vi "选择条件，选择函数的 练习.vi"() -> ()   [LabVIEW 2023]
panel:
  out "选择条件运行时间":dbl
  out "选择函数运行时间":dbl
  out "s? t:f":dbl
  in  "String 3":string
  out "Numeric 2":dbl
  in  "String 2":string
  out "x*y":dbl
  in  "stop":bool
  out "时间长度":dbl
  out "迭代次数":i32
  in  "Numeric":i32
  # "选择条件，选择函数的 练习"
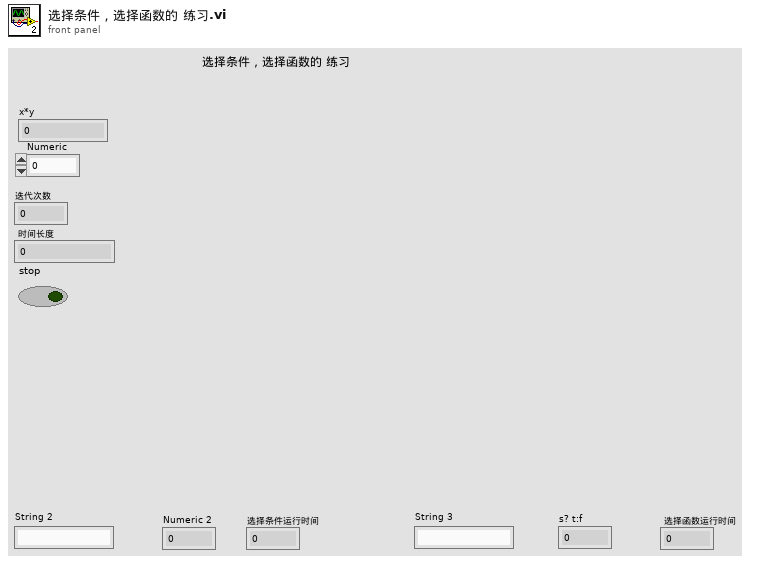
[diagram p1: front panel]
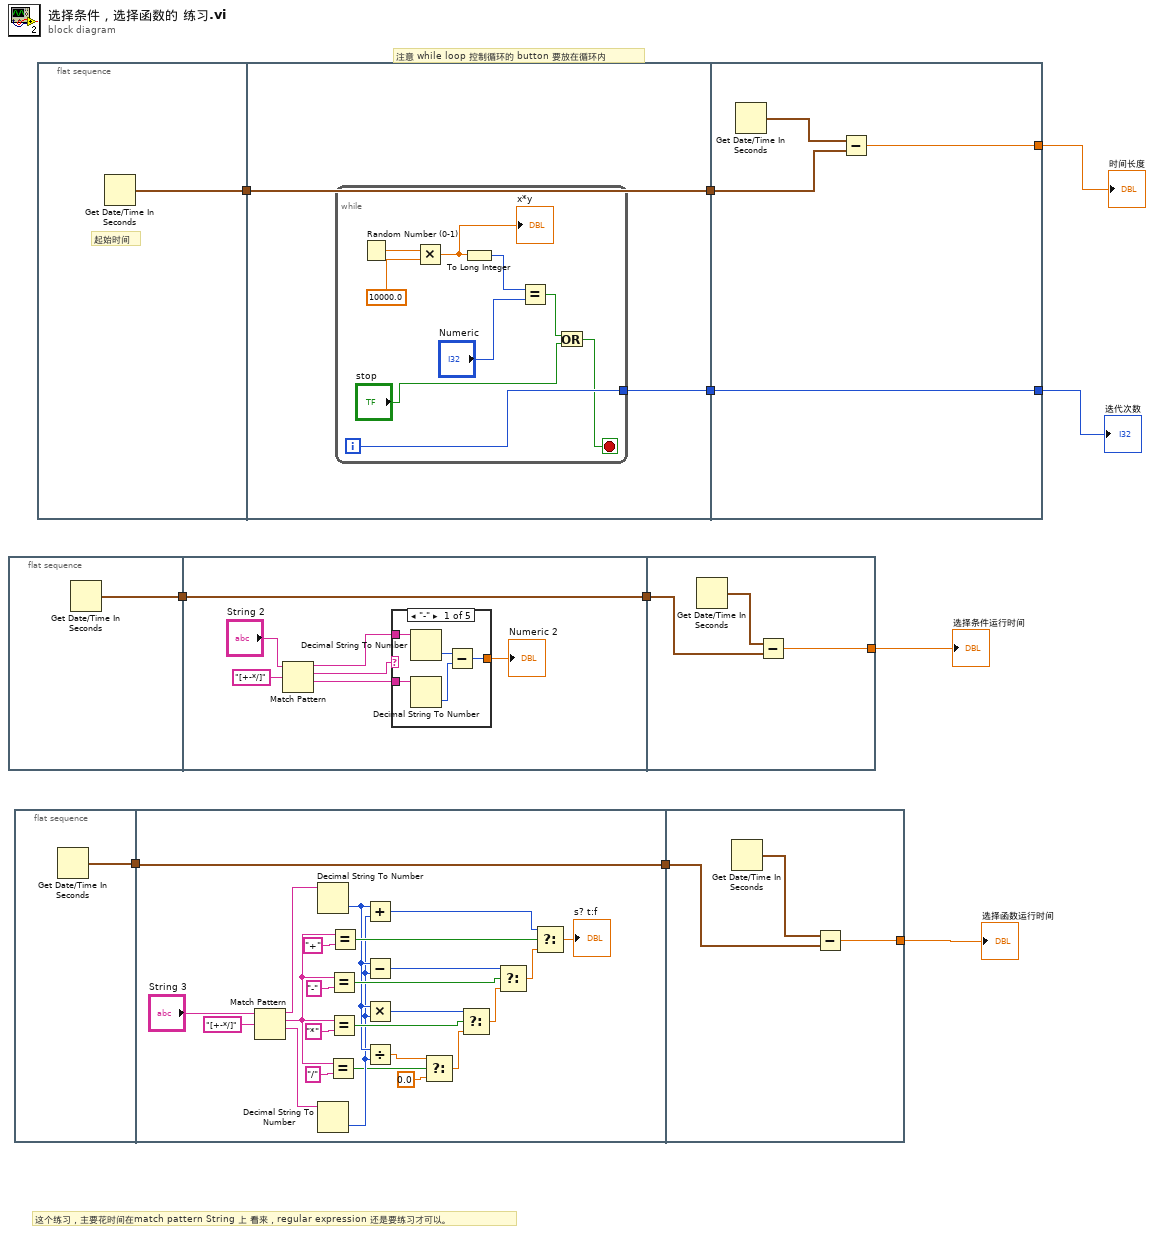
[diagram p0: block diagram]
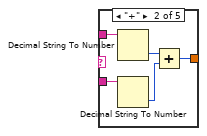
[diagram p2: hidden frame]
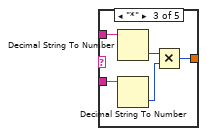
[diagram p3: hidden frame]
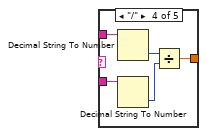
[diagram p4: hidden frame]
diagram:
  # "这个练习，主要花时间在match pattern String 上 看来，regular expression 还是要练习才可以。"
  # "注意 while loop 控制循环的 button 要放在循环内"
  n1 = flat-sequence {
    tunnel: [w12] -> w6
    tunnel: w6 -> [w13]
    tunnel: [w13] -> w2
    tunnel: w2 -> [w41]
    tunnel: [w40] -> w1
    frame #0 {
      n2 = Get Date/Time In Seconds() -> (seconds since 1Jan1904=w12:timestamp)
    }
    frame #1 {
      n3 = Match Pattern(string="String 2", regular expression="[+-*/]") -> (before substring=w16:string, match substring=w17:string, after substring=w15:string)  [unwired: 1 in, 1 out]
      n4 = case shown="\"-\"" w17 {
        tunnel: w16 -> [w24 w29 w34 w39 _]
        tunnel: w15 -> [w23 w28 w33 w38 _]
        tunnel: [w20 w25 w30 w35 _] -> w14
        frame "-" {
          n5 = Decimal String To Number(string=w24) -> (number=w22:i32)  [unwired: 2 in, 1 out]
          n6 = Decimal String To Number(string=w23) -> (number=w21:i32)  [unwired: 2 in, 1 out]
          n7 = Subtract(x=w22, y=w21) -> (x-y=w20:i32)
        }
        frame "+" {
          n8 = Decimal String To Number(string=w29) -> (number=w27:i32)  [unwired: 2 in, 1 out]
          n9 = Decimal String To Number(string=w28) -> (number=w26:i32)  [unwired: 2 in, 1 out]
          n10 = Add(x=w27, y=w26) -> (x+y=w25:i32)
        }
        frame "*" {
          n11 = Decimal String To Number(string=w34) -> (number=w32:i32)  [unwired: 2 in, 1 out]
          n12 = Decimal String To Number(string=w33) -> (number=w31:i32)  [unwired: 2 in, 1 out]
          n13 = Multiply(x=w32, y=w31) -> (x*y=w30:i32)
        }
        frame "/" {
          n14 = Decimal String To Number(string=w39) -> (number=w37:i32)  [unwired: 2 in, 1 out]
          n15 = Decimal String To Number(string=w38) -> (number=w36:i32)  [unwired: 2 in, 1 out]
          n16 = Divide(x=w37, y=w36) -> (x/y=w35:dbl)
        }
        frame Default {
        }
      }
      "Numeric 2" <- w14
    }
    frame #2 {
      n17 = Get Date/Time In Seconds() -> (seconds since 1Jan1904=w42:timestamp)
      n18 = Subtract(x=w42, y=w41) -> (x-y=w40:dbl)
    }
  }
  n19 = flat-sequence {
    tunnel: [w43] -> w5
    tunnel: w5 -> [w44]
    tunnel: [w44] -> w4
    tunnel: w4 -> [w70]
    tunnel: [w69] -> w3
    frame #0 {
      n20 = Get Date/Time In Seconds() -> (seconds since 1Jan1904=w43:timestamp)
    }
    frame #1 {
      n21 = Match Pattern(string="String 3", regular expression="[+-*/]") -> (before substring=w65:string, match substring=w52:string, after substring=w64:string)  [unwired: 1 in, 1 out]
      n22 = Decimal String To Number(string=w65) -> (number=w50:i32)  [unwired: 2 in, 1 out]
      n23 = Decimal String To Number(string=w64) -> (number=w49:i32)  [unwired: 2 in, 1 out]
      n24 = Equal?(x=w52, y="/") -> (x = y?=w47:bool)
      n25 = Equal?(x=w52, y="-") -> (x = y?=w59:bool)
      n26 = Equal?(x=w52, y="*") -> (x = y?=w54:bool)
      n27 = Equal?(x=w52, y="+") -> (x = y?=w63:bool)
      n28 = Add(x=w50, y=w49) -> (x+y=w62:i32)
      n29 = Subtract(x=w50, y=w49) -> (x-y=w58:i32)
      n30 = Multiply(x=w50, y=w49) -> (x*y=w55:i32)
      n31 = Divide(x=w50, y=w49) -> (x/y=w48:dbl)
      n32 = Select(t=w48, s=w47, f=0.0) -> (s? t:f=w53:dbl)
      n33 = Select(t=w55, s=w54, f=w53) -> (s? t:f=w57:dbl)
      n34 = Select(t=w58, s=w59, f=w57) -> (s? t:f=w60:dbl)
      n35 = Select(t=w62, s=w63, f=w60) -> (s? t:f=→"s? t:f":dbl)
    }
    frame #2 {
      n36 = Get Date/Time In Seconds() -> (seconds since 1Jan1904=w71:timestamp)
      n37 = Subtract(x=w71, y=w70) -> (x-y=w69:dbl)
    }
  }
  n38 = flat-sequence {
    tunnel: [w72] -> w11
    tunnel: w11 -> [w73]
    tunnel: [w74] -> w10
    tunnel: [w73] -> w8
    tunnel: [w87] -> w9
    tunnel: w10 -> [w87]
    tunnel: w8 -> [w85]
    tunnel: [w84] -> w7
    frame #0 {
      # "起始时间"
      n39 = Get Date/Time In Seconds() -> (seconds since 1Jan1904=w72:timestamp)
    }
    frame #1 {
      n40 = while {
        tunnel: [w80] -> w74
        i -> [w80]
        stop <- w78 stop-if-true
        n41 = Random Number (0-1)() -> (number: 0 to 1=w83:dbl)
        n42 = Multiply(x=w83, y=10000.0) -> (x*y=w76:dbl)
        "x*y" <- w76
        n43 = To Long Integer(number=w76) -> (32bit integer=w77:i32)
        n44 = Equal?(x=w77, y="Numeric") -> (x = y?=w79:bool)
        n45 = Or(x=w79, y="stop") -> (x .or. y?=w78:bool)
      }
    }
    frame #2 {
      n46 = Get Date/Time In Seconds() -> (seconds since 1Jan1904=w86:timestamp)
      n47 = Subtract(x=w86, y=w85) -> (x-y=w84:dbl)
    }
  }
  "迭代次数" <- w9
  "时间长度" <- w7
  "选择函数运行时间" <- w3
  "选择条件运行时间" <- w1
